vi "Configure Trigger Pattern.vi"(0 "VISA resource name":refnum<visa-resource-name>, 1 "Channel  3":u16(ring) items=["Don't Care", "High", "Low"], 2 "Level 3":dbl, 3 "Channel  4":u16(ring) items=["Don't Care", "High", "Low"], 4 "Level 4":dbl, 5 "error in (no error)":errorcluster, 6 "Channel  1":u16(ring) items=["Don't Care", "High", "Low"], 7 "Ecternal":u16(ring) items=["Don't Care", "High", "Low"], 8 "Level 1":dbl, 9 "Level EX":dbl, 10 "Channel  2":u16(ring) items=["Don't Care", "High", "Low"], 11 "State":u16(ring) items=["AND", "OR", "NAND", "NOR"], 12 "Level 2":dbl) -> (14 "VISA resource name out":refnum<visa-resource-name>, 19 "error out":errorcluster)   [LabVIEW 2018, in "LeCroy Wave Series.lvlib"]
doc: "Logic combination (AND, NAND, OR, NOR) of 5 inputs (4 channels and external trigger input). Each source can be high, low, or don't care. The High and Low level can be selected independently. Triggers at start or end of pattern.\nThis VI configures logical combination of channels for logic trigger."
uses:
  LeCroy Wave Series.lvlib
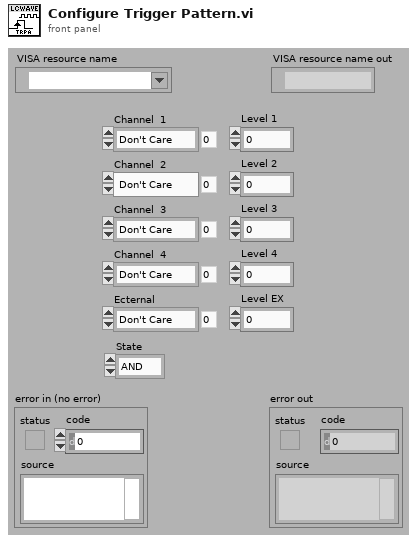
[diagram p1: front panel]
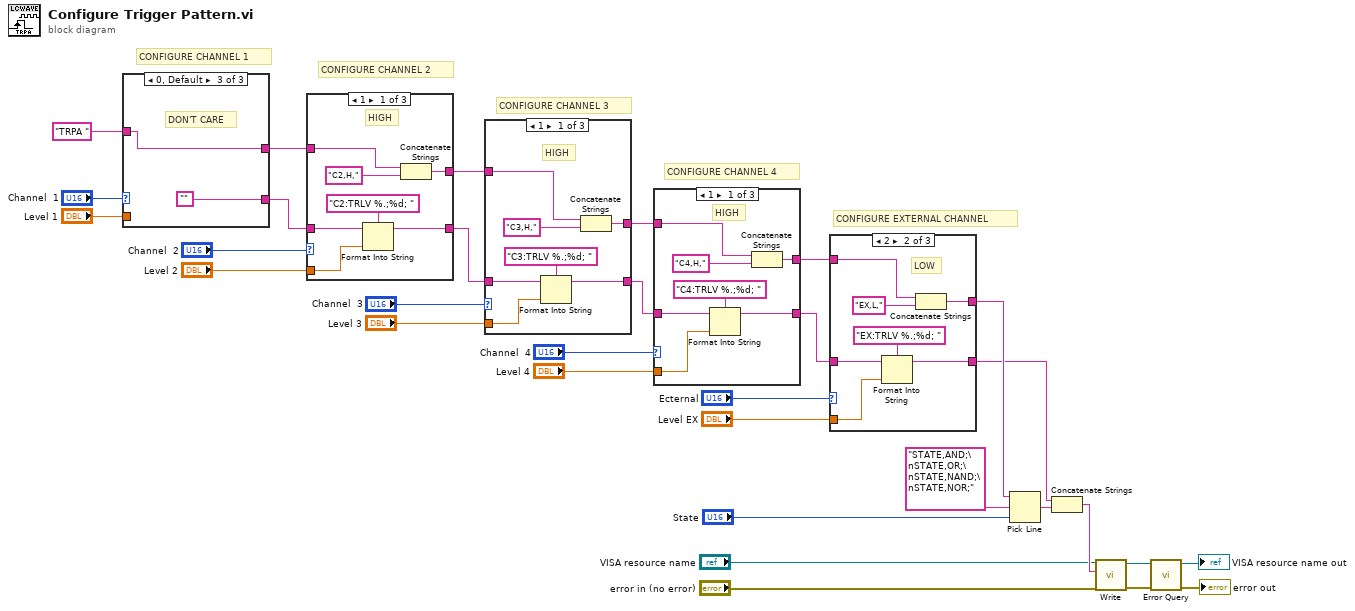
[diagram p0: block diagram]
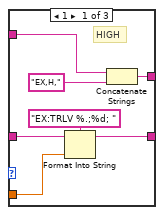
[diagram p2: hidden frame]
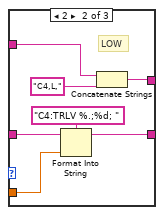
[diagram p4: hidden frame]
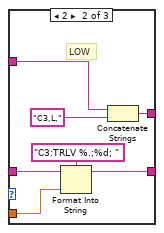
[diagram p6: hidden frame]
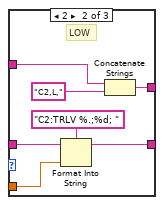
[diagram p8: hidden frame]
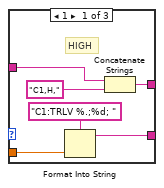
[diagram p10: hidden frame]
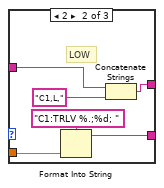
[diagram p11: hidden frame]
diagram:
  # "CONFIGURE EXTERNAL CHANNEL"
  # "CONFIGURE CHANNEL 4"
  # "CONFIGURE CHANNEL 3"
  # "CONFIGURE CHANNEL 2"
  # "CONFIGURE CHANNEL 1"
  n1 = case shown="0, Default" "Channel  1" {
    tunnel: "Level 1" -> [w37 w43 _]
    tunnel: [w34 w38 w44] -> w16
    tunnel: [w35 w41 "" ("Empty String Constant")] -> w21
    tunnel: "TRPA " -> [w32 w39 w44]
    frame 1 {
      # "HIGH"
      n2 = Format Into String(format string="C1:TRLV %.;%d; ", w37) -> (resulting string=w35:string)  [unwired: 2 in, 1 out]
      n3 = Concatenate Strings(w32, "C1,H,") -> (w34:string)
    }
    frame 2 {
      # "LOW"
      n4 = Format Into String(format string="C1:TRLV %.;%d; ", w43) -> (resulting string=w41:string)  [unwired: 2 in, 1 out]
      n5 = Concatenate Strings(w39, "C1,L,") -> (w38:string)
    }
    frame 0, Default {
      # "DON'T CARE"
    }
  }
  n6 = case shown="1" "Channel  2" {
    tunnel: "Level 2" -> [w52 w59 _]
    tunnel: [w48 w55 w60] -> w15
    tunnel: [w50 w57 w61] -> w20
    tunnel: w21 -> [w49 w56 w61]
    tunnel: w16 -> [w47 w53 w60]
    frame 1 {
      # "HIGH"
      n7 = Format Into String(format string="C2:TRLV %.;%d; ", initial string=w49, w52) -> (resulting string=w50:string)  [unwired: 1 in, 1 out]
      n8 = Concatenate Strings(w47, "C2,H,") -> (w48:string)
    }
    frame 2 {
      # "LOW"
      n9 = Format Into String(format string="C2:TRLV %.;%d; ", initial string=w56, w59) -> (resulting string=w57:string)  [unwired: 1 in, 1 out]
      n10 = Concatenate Strings(w53, "C2,L,") -> (w55:string)
    }
    frame 0, Default {
      # "DON'T CARE"
    }
  }
  n11 = case shown="1" "Channel  3" {
    tunnel: "Level 3" -> [w68 w75 _]
    tunnel: [w64 w69 w76] -> w14
    tunnel: [w66 w73 w77] -> w19
    tunnel: w20 -> [w65 w72 w77]
    tunnel: w15 -> [w63 w71 w76]
    frame 1 {
      # "HIGH"
      n12 = Format Into String(format string="C3:TRLV %.;%d; ", initial string=w65, w68) -> (resulting string=w66:string)  [unwired: 1 in, 1 out]
      n13 = Concatenate Strings(w63, "C3,H,") -> (w64:string)
    }
    frame 2 {
      # "LOW"
      n14 = Format Into String(format string="C3:TRLV %.;%d; ", initial string=w72, w75) -> (resulting string=w73:string)  [unwired: 1 in, 1 out]
      n15 = Concatenate Strings(w71, "C3,L,") -> (w69:string)
    }
    frame 0, Default {
      # "DON'T CARE"
    }
  }
  n16 = case shown="1" "Channel  4" {
    tunnel: [w80 w87 w92] -> w13
    tunnel: [w83 w90 w93] -> w18
    tunnel: "Level 4" -> [w82 w89 _]
    tunnel: w19 -> [w81 w88 w93]
    tunnel: w14 -> [w78 w86 w92]
    frame 1 {
      # "HIGH"
      n17 = Format Into String(format string="C4:TRLV %.;%d; ", initial string=w81, w82) -> (resulting string=w83:string)  [unwired: 1 in, 1 out]
      n18 = Concatenate Strings(w78, "C4,H,") -> (w80:string)
    }
    frame 2 {
      # "LOW"
      n19 = Format Into String(format string="C4:TRLV %.;%d; ", initial string=w88, w89) -> (resulting string=w90:string)  [unwired: 1 in, 1 out]
      n20 = Concatenate Strings(w86, "C4,L,") -> (w87:string)
    }
    frame 0, Default {
      # "DON'T CARE"
    }
  }
  n21 = case shown="2" "Ecternal" {
    tunnel: [w96 w101 w108] -> w10
    tunnel: [w99 w106 w109] -> w9
    tunnel: "Level EX" -> [w98 w105 _]
    tunnel: w18 -> [w97 w104 w109]
    tunnel: w13 -> [w94 w103 w108]
    frame 1 {
      # "HIGH"
      n22 = Format Into String(format string="EX:TRLV %.;%d; ", initial string=w97, w98) -> (resulting string=w99:string)  [unwired: 1 in, 1 out]
      n23 = Concatenate Strings(w94, "EX,H,") -> (w96:string)
    }
    frame 2 {
      # "LOW"
      n24 = Format Into String(format string="EX:TRLV %.;%d; ", initial string=w104, w105) -> (resulting string=w106:string)  [unwired: 1 in, 1 out]
      n25 = Concatenate Strings(w103, "EX,L,") -> (w101:string)
    }
    frame 0, Default {
      # "DON'T CARE"
    }
  }
  n26 = Pick Line(string ("")=w10, multi-line string="STATE,AND;\nSTATE,OR;\nSTATE,NAND;\nSTATE,NOR;", line index="State") -> (output string=w8:string)
  n27 = Concatenate Strings(w9, w8) -> (w7:string)
  n28 = call "Write.vi"("error in (no error)"="error in (no error)", "Write Buffer"=w7, "VISA resource name"="VISA resource name") -> ("error out"=w2:errorcluster, "VISA resource name out"=w4:refnum<visa-resource-name>)  [unwired: 7 in]
  n29 = call "Error Query.vi"("error in (no error)"=w2, "VISA resource name"=w4) -> ("error out"=→"error out":errorcluster, "VISA resource name out"=→"VISA resource name out":refnum<visa-resource-name>)  [unwired: 6 in, 2 out]
